vi "Tosca-Write AODO.vi"(0 "AO":dbl[][](array[numeric]), 5 "DO":bool[][](array[boolean]), 11 "error in (no error)":errorcluster) -> (15 "error out":errorcluster)   [LabVIEW 2020]
uses:
  epl-vi-lib/PXI DAQ VIs/AODO/Typedefs/AODO-Action.ctl
  PXI DAQ VIs/TDT VIs/TDT AODO VIs/Typedefs/TDT-AODO-Action.ctl
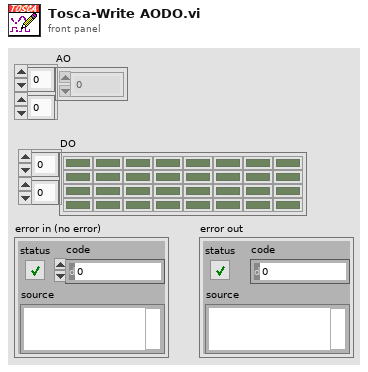
[diagram p1: front panel]
types:
  T1 = typedef "AODO-Action.ctl" = enum16{"Configure", "Initialize", "Start", "Write", "Clean up", "Init & Start", "Config & Test", "Position", "Set AO Gains", "Zero"}
  T2 = typedef "TDT-AODO-Action.ctl" = enum16{"Configure", "Initialize", "Start", "Stop", "Write", "Clean up", "Space available"}
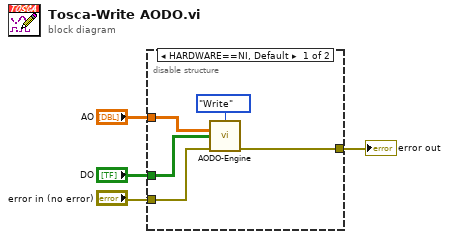
[diagram p0: block diagram]
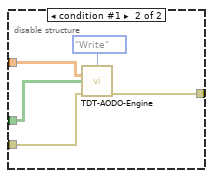
[diagram p2: hidden frame]
diagram:
  n1 = disable-structure shown="HARDWARE==NI, Default" {
    disable-tunnel: [w9 w10] -> w4
    disable-tunnel: "DO" -> [w7 w12]
    disable-tunnel: "AO" -> [w6 w13]
    disable-tunnel: "error in (no error)" -> [w5 w11]
    frame condition #0 (active) {
      n2 = call "AODO-Engine.vi"("Action"=AODO-Action."Write", "AO"=w6, "DO"=w7, "error in (no error)"=w5) -> ("error out"=w9:errorcluster)  [unwired: 10 in, 1 out]
    }
    frame condition #1 {
      n3 = call "TDT-AODO-Engine.vi"("Action"=TDT-AODO-Action."Write", "AO"=w13, "DO"=w12, "error in (no error)"=w11) -> ("error out"=w10:errorcluster)  [unwired: 9 in, 2 out]
    }
  }
  "error out" <- w4
